vi "Set Control.vi"(8 "error in (no error)":errorcluster, 9 "Output #":i32=1, 10 "Control":T1, 11 "LakeShore T Controller Driver in":refnum<class "LakeShore T Controller Driver.lvclass">) -> (0 "error out":errorcluster, 3 "LakeShore T Controller Driver out":refnum<class "LakeShore T Controller Driver.lvclass">)   [LabVIEW 2021, in "LakeShore T Controller Driver.lvclass"]
uses:
  Temperature Controller/Controls/Control Mode.ctl
  LakeShore T Controller Driver.lvclass
  LakeShore T Controller Driver.lvclass/LakeShore T Controller Driver.ctl
  LakeShore340/LakeShore340 Mode.ctl
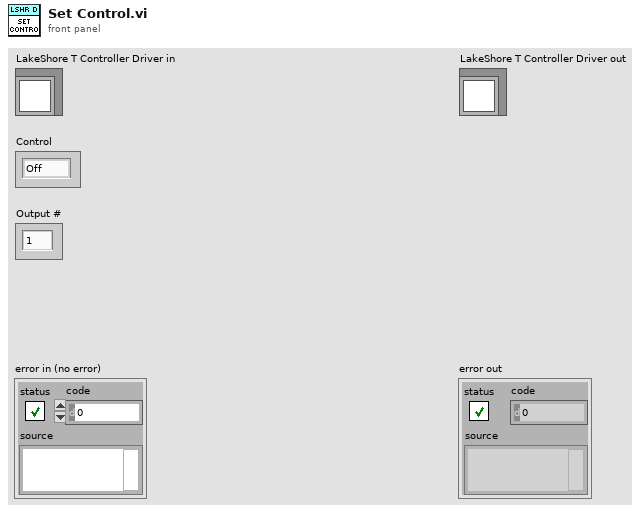
[diagram p1: front panel]
types:
  T1 = typedef "Control Mode.ctl" = enum16{"Off", "PID", "Ramp", "Manual", "Table"}
  T2 = typedef "LakeShore340 Mode.ctl" = enum16{"Off", "Manual PID", "Zone", "Open loop", "AutoTune PID", "AutoTune PI", "AutoTune P"}
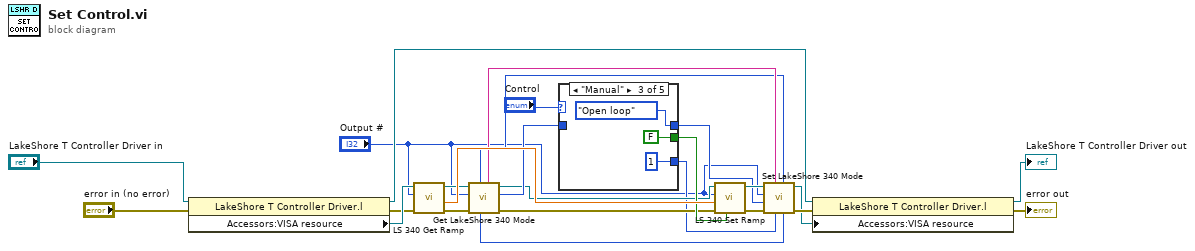
[diagram p0: block diagram]
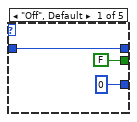
[diagram p2: hidden frame]
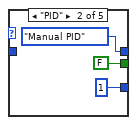
[diagram p3: hidden frame]
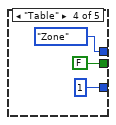
[diagram p4: hidden frame]
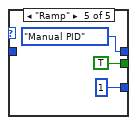
[diagram p5: hidden frame]
diagram:
  n1 = property class="LakeShore T Controller Driver.l"(reference="LakeShore T Controller Driver in", error in="error in (no error)") -> (reference out=w13:refnum<class "LakeShore T Controller Driver.lvclass">, error out=w7:errorcluster, "Accessors:VISA resource"=w24:refnum<visa-resource-name>)
  n2 = call "LS 340 Get Ramp.vi"("error in (no error)"=w7, "Output #"="Output #", "VISA resource name"=w24) -> ("error out"=w15:errorcluster, "Ramp rate, K/min"=w22:dbl, "VISA Resource Name Out"=w20:refnum<visa-resource-name>)  [unwired: 5 in, 1 out]
  n3 = call "Get LakeShore 340 Mode.vi"("error in (no error)"=w15, "Output #"="Output #", "VISA Resource Name"=w20) -> ("error out"=w6:errorcluster, "Lake shore mode"=w19:T2, "VISA Resource Name Out"=w14:refnum<visa-resource-name>, "Input chan"=w4:string, "powerup enable"=w3:i32, "units"=w2:i32)  [unwired: 2 in, 1 out]
  n4 = case shown="\"Manual\"" "Control" {
    tunnel: [FALSE ("Ramp on") FALSE ("Ramp on") FALSE ("Ramp on") FALSE ("Ramp on") TRUE ("Ramp on")] -> w21
    tunnel: w19 -> [w27 _ _ _ _]
    tunnel: [w27 LakeShore340_Mode."Manual PID" ("Lake shore mode") LakeShore340_Mode."Open loop" ("Lake shore mode") LakeShore340_Mode."Zone" ("Lake shore mode") LakeShore340_Mode."Manual PID" ("Lake shore mode")] -> w16
    tunnel: [0 ("on/off") 1 ("on/off") 1 ("on/off") 1 ("on/off") 1 ("on/off")] -> w5
    frame "Off", Default {
    }
    frame "PID" {
    }
    frame "Manual" {
    }
    frame "Table" {
    }
    frame "Ramp" {
    }
  }
  n5 = call "LS 340 Set Ramp.vi"("Ramp on"=w21, "error in (no error)"=w6, "Ramp rate, K/min"=w22, "Output #"="Output #", "VISA resource name"=w14) -> ("error out"=w18:errorcluster, "VISA Resource Name Out"=w17:refnum<visa-resource-name>)  [unwired: 5 in]
  n6 = call "Set LakeShore 340 Mode.vi"("enable after power cycle"=w3, "units"=w2, "on/off"=w5, "Input chan"=w4, "error in (no error)"=w18, "Lake shore mode"=w16, "Output #"="Output #", "VISA Resource Name"=w17) -> ("error out"=w11:errorcluster, "VISA Resource Name Out"=w9:refnum<visa-resource-name>)  [unwired: 2 in]
  n7 = property class="LakeShore T Controller Driver.l"(reference=w13, error in=w11, "Accessors:VISA resource"=w9) -> (reference out=→"LakeShore T Controller Driver out":refnum<class "LakeShore T Controller Driver.lvclass">, error out=→"error out":errorcluster)
